vi "Periodic Tasks.vi"(8 "error in":errorcluster) -> ()   [LabVIEW 2015]
doc: "This VI runs in parallel to other tasks. It can contain as many user-defined periodic loops as you need. These can carry out PID or other sorts of timed response."
uses:
  <vilib>/Rock Robotics/WPI/DriverStation/WPI_DriverStationRobotMode2.ctl
  <vilib>/Rock Robotics/WPI/Utilities/WPI_GetSetVariantRefNum.vi
  Robot Global Data.vi
  <vilib>/Rock Robotics/Network Tables/NT Write String Array.vi
  <vilib>/Rock Robotics/Network Tables/NT Write Numeric Array.vi
  <vilib>/Rock Robotics/Network Tables/NT Write Boolean Array.vi
  NAVx-MXP/navX-MXP IMU.lvlib
panel:
  out "Valid? 2":bool
  out "Valid?":bool
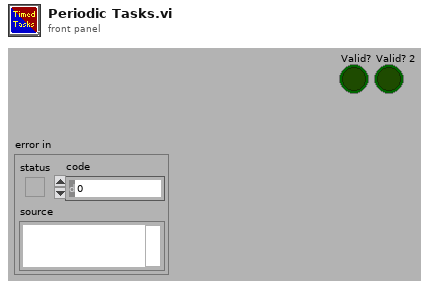
[diagram p1: front panel]
types:
  T1 = typedef "WPI_JoystickDevRef.ctl" = cluster{"Device":T2}
  T2 = typedef "WPI_JoystickDeviceEnum.ctl" = enum16{"USB 0", "USB 1", "USB 2", "USB 3", "USB 4", "USB 5"}
  T3 = typedef "WPI_RobotDriveDevRef.ctl" = cluster{"DevStatus":errorcluster, "Motors[]":T4[], "Square Inputs":bool, "Max Output":dbl}
  T4 = typedef "WPI_MotorControlDeviceRef.ctl" = cluster{"DeviceStatus":errorcluster, "Type":T5, "PWM":cluster{"PWM Channel":T6, "DeadBand":T7}, "CAN":cluster{"Device Number":u8, "Control Mode":T8, "Semaphore":T9, "Max Vout":dbl, "TalonSRX Control Mode":T10}, "Invert":bool}
  T5 = typedef "WPI_MotorControlType.ctl" = enum16{"PWM", "CAN", "CANTalonSRX"}
  T6 = typedef "FPGA_DIOPWMChannel.ctl" = enum8{"PWM 0", "PWM 1", "PWM 2", "PWM 3", "PWM 4", "PWM 5", "PWM 6", "PWM 7", "PWM 8", "PWM 9", "PWM MXP 0", "PWM MXP 1", "PWM MXP 2", "PWM MXP 3", "PWM MXP 4", "PWM MXP 5", "PWM MXP 6", "PWM MXP 7", "PWM MXP 8", "PWM MXP 9", "Invalid"}
  T7 = typedef "WPI_PWMDeadband.ctl" = cluster{"Name":string, "maxPositivePwm":i32, "minPositivePwm":i32, "centerPwm":i32, "maxNegativePwm":i32, "minNegativePwm":i32, "angularRange":u16}
  T8 = typedef "WPI_CANJaguar_ControlMode.ctl" = enum8{"Percent VBus", "Current", "Speed", "Position", "Voltage"}
  T9 = typedef "Semaphore RefNum" = refnum<k1>
  T10 = typedef "WPI_CANTalonSRX_APIControlMode.ctl" = enum8{"Percent VBus", "Speed", "Position", "Slave", "Unchanged / Invalid", "Voltage Compensation", "Current"}
  T11 = typedef "WPI_GyroDevRef.ctl" = cluster{"DevStatus":errorcluster, "Analog Channel":T12, "Offset":dbl, "Gain (VoltsPerDegree/Second)":dbl}
  T12 = typedef "FPGA_AIChannel.ctl" = enum8{"AI 0", "AI 1", "AI 2", "AI 3", "AI MXP 0", "AI MXP 1", "AI MXP 2", "AI MXP 3", "Invalid"}
  T13 = typedef "navX-MXP IMU.lvlib/navX Device TypeDef.ctl" = cluster{"navX Interface Protocol":T14, "navX Interface Protocol TypeDefs":cluster{"SPIDevRef":T15, "I2CDevRef":T17}, "navX System Information":cluster{"Board Information":T19, "Status":T22, "Offsets":T26, "LastSampleTimestamp":dbl, "LastSampleValid":bool}, "navX Common Information":cluster{"Update Rate (4Hz-60Hz)":T27, "refnum name":string, "error":errorcluster, "LastSampleFPGATimestamp":dbl}}
  T14 = typedef "navX-MXP IMU.lvlib/navX Interface Protocol.ctl" = enum16{"SPI", "I2C", "SERIAL"}
  T15 = typedef "WPI_SPIDevRef.ctl" = cluster{"DevStatus":errorcluster, "Handle":i32, "SPI Bus":T16}
  T16 = typedef "spi_bus.ctl" = enum16{"SPI On-Board, CS0", "SPI On-Board, CS1", "SPI On-Board, CS2", "SPI On-Board, CS3", "SPI MXP", "Invalid"}
  T17 = typedef "WPI_I2CDevRef.ctl" = cluster{"DevStatus":errorcluster, "Device Address":u8, "Handle":i32, "I2C Bus":T18}
  T18 = typedef "i2c_bus.ctl" = enum16{"I2C On-Board", "I2C MXP", "Invalid"}
  T19 = typedef "navX-MXP IMU.lvlib/navX Board Information.ctl" = cluster{"WhoAmI (50 | 0x32)":u8, "Board Revision":u8, "Firmware Major Version":u8, "Firmware Minor Version":u8, "NAVX_BOARD_CAPABILITY":T20, "NAVX_BOARD_YAW_AXIS":T21}
  T20 = typedef "navX-MXP IMU.lvlib/navX NAVX_BOARD_CAPABILITY.ctl" = cluster{"OMNIMOUNT":bool, "YAW_RESET":bool, "VEL_AND_DISP":bool}
  T21 = typedef "navX-MXP IMU.lvlib/navX NAVX_BOARD_YAW_AXIS.ctl" = cluster{"BOARD_YAW_AXIS_UP":bool, "BOARD_YAW_AXIS":u8}
  T22 = typedef "navX-MXP IMU.lvlib/navX Status Data.ctl" = cluster{"Update Rate Hz":u8, "Accelerometer Full-Scale Range":u8, "Gyro Full-Scale Range":u16, "NAVX_OP_STATUS":T23, "NAVX_CAL_STATUS":T24, "NAVX_SELFTEST_STATUS":u8, "NAVX_SENSOR_STATUS":T25}
  T23 = typedef "navX-MXP IMU.lvlib/navX NAVX_OP_STATUS.ctl" = u8
  T24 = typedef "navX-MXP IMU.lvlib/navX NAVX_CAL_STATUS.ctl" = u8
  T25 = typedef "navX-MXP IMU.lvlib/navX NAVX_SENSOR_STATUS.ctl" = cluster{"MOVING":bool, "YAW_STABLE":bool, "MAG_DISTURBANCE":bool, "ALTITUDE_VALID":bool, "SEALEVEL_PRESS_SET":bool, "FUSED_HEADING_VALID":bool}
  T26 = typedef "navX-MXP IMU.lvlib/navX Offsets Data.ctl" = cluster{"Yaw":dbl, "Quat W":dbl, "Quat X":dbl, "Quat Y":dbl, "Quat Z":dbl}
  T27 = typedef "navX-MXP IMU.lvlib/navX Update Rate.ctl" = u8
  T28 = cluster{"JoystickDevRef":T1, "RobotDriveDevRef":T3}
  T29 = typedef "WPI_DriverStationRobotMode2.ctl" = enum16{"Autonomous Disabled", "Autonomous Enabled", "Teleop Disabled", "Teleop Enabled", "Disconnected", "Finish", "Test Disabled", "Test Enabled", "Emergency Stopped"}
  T30 = enum16{"CW_Fast", "CW_Slow", "CCW_Fast", "CCW_Slow", "Straight", "WaitingForStraight", "Rotate_Move"}
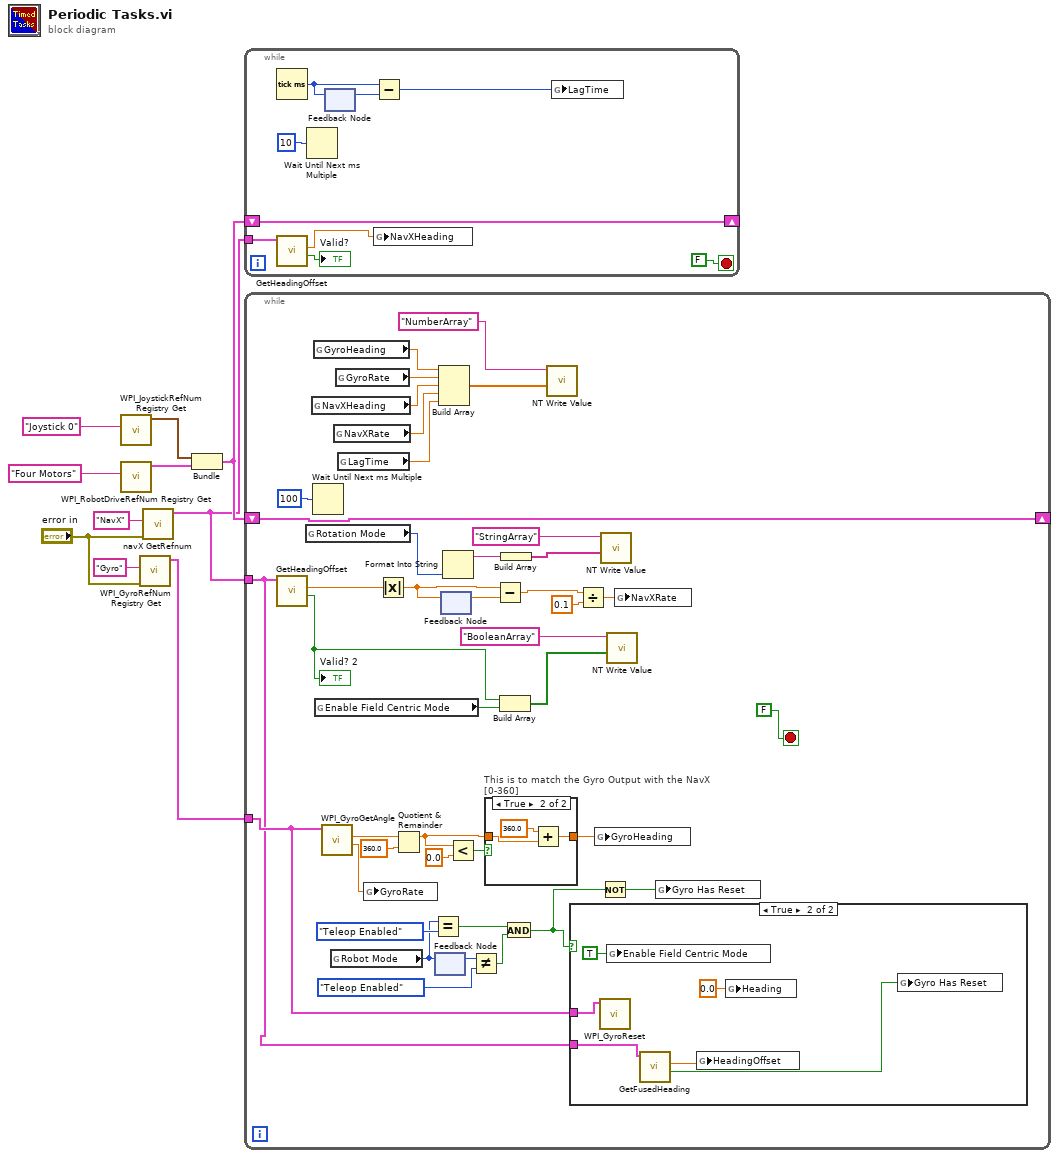
[diagram p0: block diagram]
diagram:
  n1 = call <vilib>:"WPI_JoystickRefNum Registry Get.vi"("refnum name"="Joystick 0") -> ("JoystickDevRef"=w8:T1)  [unwired: 1 in, 9 out]
  n2 = call <vilib>:"WPI_RobotDriveRefNum Registry Get.vi"("refnum name"="Four Motors") -> ("RobotDriveDevRef"=w7:T3)  [unwired: 1 in, 9 out]
  n3 = call <vilib>:"WPI_GyroRefNum Registry Get.vi"("error in (no error)"="error in", "refnum name"="Gyro") -> ("GyroDevRef"=w1:T11)  [unwired: 8 in, 1 out]
  n4 = call "navX GetRefnum.vi"("error in (no error)"="error in", "refnum name"="NavX") -> ("navX Device TypeDef"=w2:T13)  [unwired: 8 in, 1 out]
  n5 = Bundle("JoystickDevRef"=w8, "RobotDriveDevRef"=w7) -> (w6:T28)  [unwired: 1 out]
  n6 = while {
    shift-right: [w17] -> _
    shift-left: w6 -> [w17]
    tunnel: w2 -> [w14]
    stop <- FALSE stop-if-true
    n7 = Tick Count (ms)() -> (millisecond timer value=w16:u32)
    n8 = call "GetHeadingOffset.vi"("navX Device TypeDef"=w14) -> ("Valid?"=→"Valid?":bool, "Offset Heading"=w12:dbl)  [unwired: 8 in, 1 out]
    n9 = Wait Until Next ms Multiple(millisecond multiple=u32 10 ("milliseconds to wait")) -> ()  [unwired: 1 out]
    n10 = feedback-in #1(w16) -> ()
    n11 = feedback #1() -> (w15:u32)  [unwired: 1 in]
    n12 = Subtract(x=w16, y=w15) -> (x-y=w11:u32)
    n13 = global write "Robot Global Data.vi" "NavXHeading"(w12) -> ()
    n14 = global write "Robot Global Data.vi" "LagTime"(w11) -> ()
  }
  n15 = while {
    shift-right: [w58] -> _
    shift-left: w6 -> [w58]
    tunnel: w2 -> [w24]
    tunnel: w1 -> [w25]
    stop <- FALSE stop-if-true
    n16 = call "GetHeadingOffset.vi"("navX Device TypeDef"=w24) -> ("Valid?"=w46:bool, "Offset Heading"=w23:dbl)  [unwired: 8 in, 1 out]
    "Valid? 2" <- w46
    n17 = global read "Robot Global Data.vi" "Rotation Mode"() -> (w42:T30)
    n18 = global read "Robot Global Data.vi" "NavXHeading"() -> (w50:dbl)
    n19 = Wait Until Next ms Multiple(millisecond multiple=u32 100 ("milliseconds to wait")) -> ()  [unwired: 1 out]
    n20 = global read "Robot Global Data.vi" "GyroHeading"() -> (w53:dbl)
    n21 = global read "Robot Global Data.vi" "Enable Field Centric Mode"() -> (w45:bool)
    n22 = call <vilib>:"WPI_GyroGetAngle.vi"("GyroDevRef"=w25) -> ("Angular Rate"=w38:dbl, "Angle"=w37:dbl)  [unwired: 7 in, 2 out]
    n23 = global read "Robot Global Data.vi" "Robot Mode"() -> (w29:T29)
    n24 = global read "Robot Global Data.vi" "NavXRate"() -> (w48:dbl)
    n25 = global read "Robot Global Data.vi" "GyroRate"() -> (w51:dbl)
    n26 = global read "Robot Global Data.vi" "LagTime"() -> (w44:dbl)
    n27 = global write "Robot Global Data.vi" "GyroRate"(w38) -> ()
    n28 = Absolute Value(x=w23) -> (abs(x)=w20:dbl)
    n29 = Quotient & Remainder(x=w37, y=360.0) -> (x-y*floor(x/y)=w32:dbl)  [unwired: 1 out]
    n30 = Equal?(x=w29, y=WPI_DriverStationRobotMode2."Teleop Enabled") -> (x = y?=w30:bool)
    n31 = feedback-in #2(w29) -> ()
    n32 = feedback #2() -> (w28:T29)  [unwired: 1 in]
    n33 = Build Array(w53, w51, w50, w48, w44) -> (w52:dbl[])
    n34 = feedback #3() -> (w55:dbl)  [unwired: 1 in]
    n35 = feedback-in #3(w20) -> ()
    n36 = Format Into String(w42) -> (resulting string=w41:string)  [unwired: 3 in, 1 out]
    n37 = Less?(x=w32, y=0.0) -> (x < y?=w34:bool)
    n38 = Not Equal?(x=w28, y=WPI_DriverStationRobotMode2."Teleop Enabled") -> (x != y?=w26:bool)
    n39 = case "This is to match the Gyro Output with the NavX [0-360]" shown="True" w34 {
      tunnel: [w67 w70] -> w35
      tunnel: w32 -> [w67 w68]
      frame False {
      }
      frame True {
        n40 = Add(x=360.0, y=w68) -> (x+y=w70:dbl)
      }
    }
    n41 = Subtract(x=w20, y=w55) -> (x-y=w56:dbl)
    n42 = Build Array(w46, w45) -> (w47:bool[])
    n43 = Build Array(w41) -> (w40:string[])
    n44 = And(x=w30, y=w26) -> (x .and. y?=w21:bool)
    n45 = call-poly <vilib>:"NT Write Value.vi"("Numeric Array"=w52, "Name"="NumberArray") -> ()  [unwired: 9 in, 1 out]
    n46 = case shown="True" w21 {
      tunnel: w25 -> [_ w66]
      tunnel: w24 -> [_ w63]
      frame False {
      }
      frame True {
        n47 = call <vilib>:"WPI_GyroReset.vi"("GyroDevRef"=w66) -> ()  [unwired: 9 in, 2 out]
        n48 = global write "Robot Global Data.vi" "Enable Field Centric Mode"(TRUE ("Enable Field Centric Mode")) -> ()
        n49 = call "GetFusedHeading.vi"("navX Device TypeDef"=w63) -> ("Valid?"=w61:bool, "Fused Heading"=w62:dbl)  [unwired: 8 in, 1 out]
        n50 = global write "Robot Global Data.vi" "HeadingOffset"(w62) -> ()
        n51 = global write "Robot Global Data.vi" "Heading"(0.0 ("Heading")) -> ()
        n52 = global write "Robot Global Data.vi" "Gyro Has Reset"(w61) -> ()
      }
    }
    n53 = Divide(x=w56, y=0.1) -> (x/y=w57:dbl)
    n54 = global write "Robot Global Data.vi" "GyroHeading"(w35) -> ()
    n55 = Not(x=w21) -> (.not. x?=w22:bool)
    n56 = call-poly <vilib>:"NT Write Value.vi"("String Array"=w40, "Name"="StringArray") -> ()  [unwired: 9 in, 1 out]
    n57 = call-poly <vilib>:"NT Write Value.vi"("Boolean Array"=w47, "Name"="BooleanArray") -> ()  [unwired: 9 in, 1 out]
    n58 = global write "Robot Global Data.vi" "NavXRate"(w57) -> ()
    n59 = global write "Robot Global Data.vi" "Gyro Has Reset"(w22) -> ()
  }
